vi "CRYGet SaveAsFileName.vi"(0 "Start path":path, 1 "TitleName":string="Save As", 2 "ButtonName":string="Save", 5 "default name":string, 7 "pattern (all files)":string="*.cre", 9 "pattern label":string, 11 "error in":errorcluster, 12 "Category Name":string, 13 "Enum":enum16{"Yes_No_Cancel", "Replace_Append_Cancel"}(ring)) -> (4 "Path":path, 6 "Which Button?":T1(ring), 8 "Is Replace?":bool, 10 "stripped path":path, 15 "error out":errorcluster)   [LabVIEW 2013]
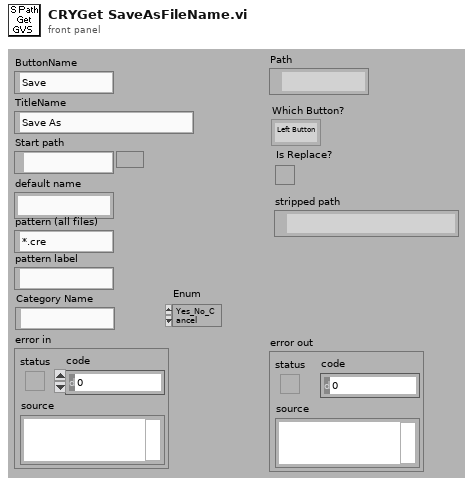
[diagram p1: front panel]
types:
  T1 = enum16{"Left Button", "Center Button", "Right Button", "Window Close"}
  T2 = enum16{"OK", "Yes", "YesNo", "YesNoCancel", "ReplaceAppend"}
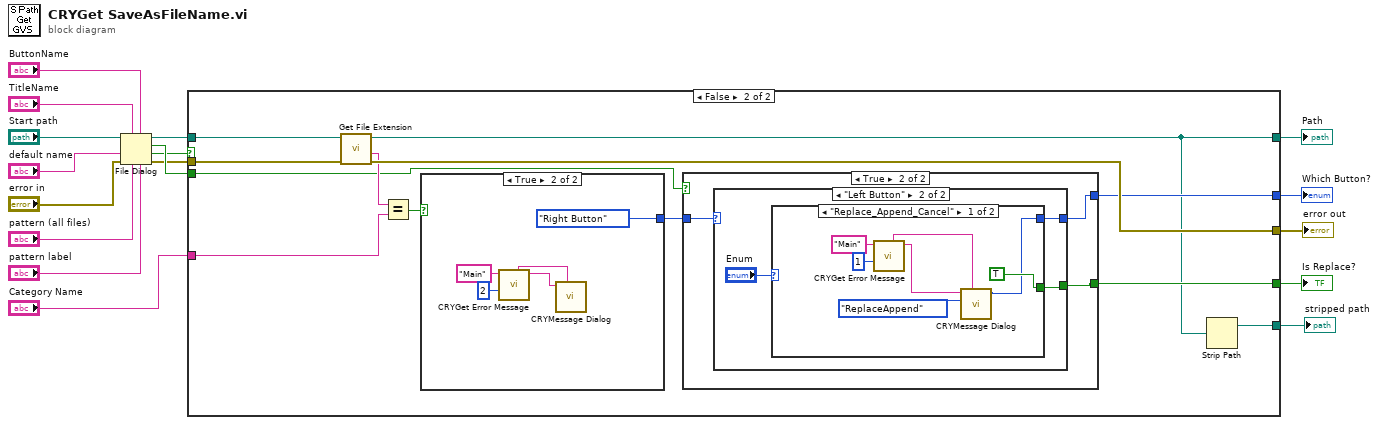
[diagram p0: block diagram]
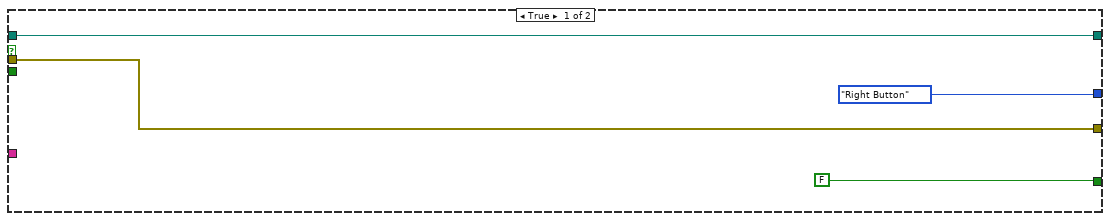
[diagram p2: hidden frame]
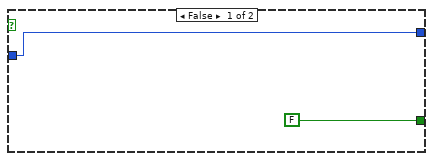
[diagram p3: hidden frame]
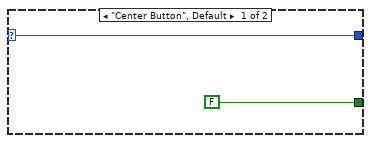
[diagram p4: hidden frame]
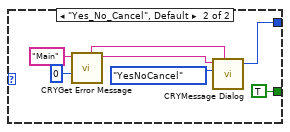
[diagram p5: hidden frame]
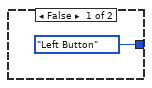
[diagram p6: hidden frame]
diagram:
  n1 = File Dialog(4:"pattern label", 5:"ButtonName", 6:"pattern (all files)", 7:"TitleName", 8:"error in", 9:"default name", 11:"Start path") -> (0:w6:errorcluster, 1:w12:bool, 2:w13:bool, 3:w15:path)
  n2 = case shown="False" w12 {
    tunnel: w15 -> [w21 w33]
    tunnel: w13 -> [_ w28]
    tunnel: "Category Name" -> [_ w22]
    tunnel: [w21 w24] -> w7
    tunnel: w6 -> [w20 w32]
    tunnel: [w20 w31] -> w5
    tunnel: [T1."Right Button" ("Which Button?") w26] -> w3
    tunnel: [FALSE ("Is Replace?") w25] -> w2
    tunnel: [_ w23] -> w1
    frame True {
    }
    frame False {
      n3 = call <vilib>:"Get File Extension.vi"("error in (no error)"=w32, "file"=w33) -> ("error out"=w31:errorcluster, "filename without extension"=w29:string, "dup file"=w24:path)  [unwired: 7 out]
      n4 = Equal?(x=w29, y=w22) -> (x = y?=w30:bool)
      n5 = case shown="True" w30 {
        tunnel: [T1."Left Button" ("Which Button?") T1."Right Button" ("Which Button?")] -> w27
        frame False {
        }
        frame True {
          n6 = call "CRYGet Error Message.vi"("Error No"=2, "Kind"="Main") -> ("Message"=w59:string, "Window Title"=w60:string)  [unwired: 4 in, 4 out]
          n7 = call "CRYMessage Dialog.vi"("Window Title"=w60, "Message Content"=w59) -> ()  [unwired: 8 in, 2 out]
        }
      }
      n8 = case shown="True" w28 {
        tunnel: [w35 w38] -> w26
        tunnel: w27 -> [w35 w37]
        tunnel: [FALSE ("Is Replace?") w36] -> w25
        frame False {
        }
        frame True {
          n9 = case shown="\"Left Button\"" w37 {
            selector: w37 -> [w40 _]
            tunnel: [w40 w43] -> w38
            tunnel: [FALSE ("Is Replace?") w41] -> w36
            frame "Center Button", Default {
            }
            frame "Left Button" {
              n10 = case shown="\"Replace_Append_Cancel\"" "Enum" {
                tunnel: [w44 w54] -> w43
                tunnel: [TRUE ("Is Replace?") TRUE ("Is Replace?")] -> w41
                frame "Replace_Append_Cancel" {
                  n11 = call "CRYGet Error Message.vi"("Error No"=1, "Kind"="Main") -> ("Message"=w46:string, "Window Title"=w47:string)  [unwired: 4 in, 4 out]
                  n12 = call "CRYMessage Dialog.vi"("Window Title"=w47, "YesNoCancel"=T2."ReplaceAppend", "Message Content"=w46) -> ("Which Button?"=w44:T1)  [unwired: 7 in, 1 out]
                }
                frame "Yes_No_Cancel", Default {
                  n13 = call "CRYGet Error Message.vi"("Error No"=0, "Kind"="Main") -> ("Message"=w52:string, "Window Title"=w53:string)  [unwired: 4 in, 4 out]
                  n14 = call "CRYMessage Dialog.vi"("Window Title"=w53, "YesNoCancel"=T2."YesNoCancel", "Message Content"=w52) -> ("Which Button?"=w54:T1)  [unwired: 7 in, 1 out]
                }
              }
            }
          }
        }
      }
      n15 = Strip Path(path=w24) -> (stripped path=w23:path)  [unwired: 1 out]
    }
  }
  "Path" <- w7
  "error out" <- w5
  "Which Button?" <- w3
  "Is Replace?" <- w2
  "stripped path" <- w1
